vi "Subvi probes.vi"   [LabVIEW 2017]
uses:
  <vilib>/Platform/TimedLoop/XDataNode/timing_clust.ctl
  <vilib>/Platform/TimedLoop/XDataNode/nitl_modes.ctl
  <vilib>/Platform/TimedLoop/XDataNode/wakeup.ctl
  <vilib>/rvi/Emulation/niFpgaSctlEmulationGetInTimedLoop.vi
  <vilib>/rvi/Emulation/niFpgaEmulationReportErrorSimple.vi
  <vilib>/rvi/Emulation/niFpgaGetClockAttributes.vi
  <vilib>/rvi/Emulation/niFpgaCriticalErrorInLSC.vi
  GV DO0.vi
  GV DO1.vi
  GV DO4.vi
  GV DO2.vi
  GV DO3.vi
  GV DO5.vi
  GV DO6.vi
  GV DO7.vi
  <vilib>/rvi/eio/common/nirviEmuTemplateMethod_errors.vi
  <vilib>/Platform/TimedLoop/XDataNode/XDataNode.xnode
  <vilib>/eio/EIONode/EIONode.xnode
  <vilib>/Platform/TimedLoop/XDataNode/XDNodeRunTimeDep.lvlib
types:
  T1 = typedef "XDNodeRunTimeDep.lvlib/timing_clust.ctl" = cluster{"Expected End [f-1]":u64, "Actual End [f-1]":u64, "Finished Late? [f-1]":bool, "Expected End [i-1]":u64, "Actual End [i-1]":u64, "Finished Late? [i-1]":bool, "Expected Start [i]":u64, "Actual Start [i]":u64, "Expected Start [f]":u64, "Actual Start [f]":u64, "Source Name":string, "Structure Name":string, "Period":i64, "Deadline":i64, "Offset":i64, "Start":i64, "Priority":i32, "Timeout":i32, "Mode":T2, "Wakeup Reason":T3, "Error":errorcluster, "Source Type":string, "Secondary Source Type":string, "Global End Time":u64, "Global Start Time":u64, "Frame Duration":u64, "Iteration Duration":u64, "Assigned CPU":i32, "I/O Scan Engine Mode":u32}
  T2 = typedef "XDNodeRunTimeDep.lvlib/nitl_modes.ctl" = enum32{"No Change", "Process missed periods, maintain original phase", "Discard missed periods, maintain original phase", "Process missed periods, ignore original phase", "Discard missed periods, ignore original phase"}
  T3 = typedef "XDNodeRunTimeDep.lvlib/wakeup.ctl" = enum32{"Normal", "Aborted", "Asynchronous wakeup", "Timing source error", "Timed loop error", "Timeout"}
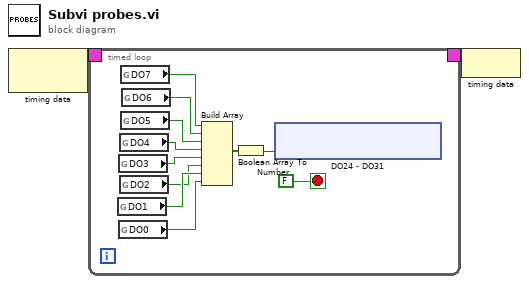
[diagram p0: block diagram]
diagram:
  n1 = node-c288() -> (w2:T1)  [unwired: 1 in]
  n2 = timed-loop {
    timing: w2 -> [_]
    timing-out: [_] -> w1
    stop <- FALSE stop-if-true
    n3 = global read "GV DO1.vi" "DO1"() -> (w11:bool)
    n4 = global read "GV DO3.vi" "DO3"() -> (w9:bool)
    n5 = global read "GV DO0.vi" "DO0"() -> (w12:bool)
    n6 = global read "GV DO4.vi" "DO4"() -> (w8:bool)
    n7 = global read "GV DO2.vi" "DO2"() -> (w10:bool)
    n8 = global read "GV DO7.vi" "DO7"() -> (w5:bool)
    n9 = global read "GV DO5.vi" "DO5"() -> (w7:bool)
    n10 = global read "GV DO6.vi" "DO6"() -> (w6:bool)
    n11 = Build Array(w5, w6, w7, w8, w9, w10, w11, w12) -> (w4:bool[])
    n12 = Boolean Array To Number(Boolean array=w4) -> (number=w3:u8)
    n13 = xnode "DO24 - DO31"("Connector0/DIOPORT3"=w3) -> ()  [unwired: 1 in, 1 out]
  }
  n14 = node-c288(w1) -> ()
